vi "Trajectory Example.vi"() -> ()   [LabVIEW 2019]
uses:
  Typedef/Trajectory.ctl
  Typedef/Trajectory State.ctl
  Geometry/Typedef/Pose2d.ctl
  Geometry/Typedef/Translation2d.ctl
  Geometry/Typedef/Rotation2d.ctl
  Typedef/Differential Drive Constants.ctl
  Typedef/Differential Drive Constraints.ctl
panel:
  in  "Constraints":T1={"maxVoltage"=10.0, "maxVelocity"=5.0, "maxAccel"=10.0}
  in  "Constants":T2={"ks"=0.2, "kv"=0.18, "ka"=0.1, "trackwidth"=1.0}
  in  "Waypoints":T3[](array[typedef])=[{"Translation2d"={"x"=0.0, "y"=0.0}, "Rotation2d"={"Theta"=0.0}}, {"Translation2d"={"x"=1.0, "y"=1.0}, "Rotation2d"={"Theta"=1.0}}, {"Translation2d"={"x"=3.0, "y"=4.0}, "Rotation2d"={"Theta"=2.0}}]
  out "states":T6
  out "XY Graph 2":cluster{dbl[], dbl[]}(graph)
  out "XY Graph":cluster{dbl[], dbl[]}[](graph)
  out "Total Time Seconds":dbl
  out "error out":errorcluster
  in  "error in (no error)":errorcluster
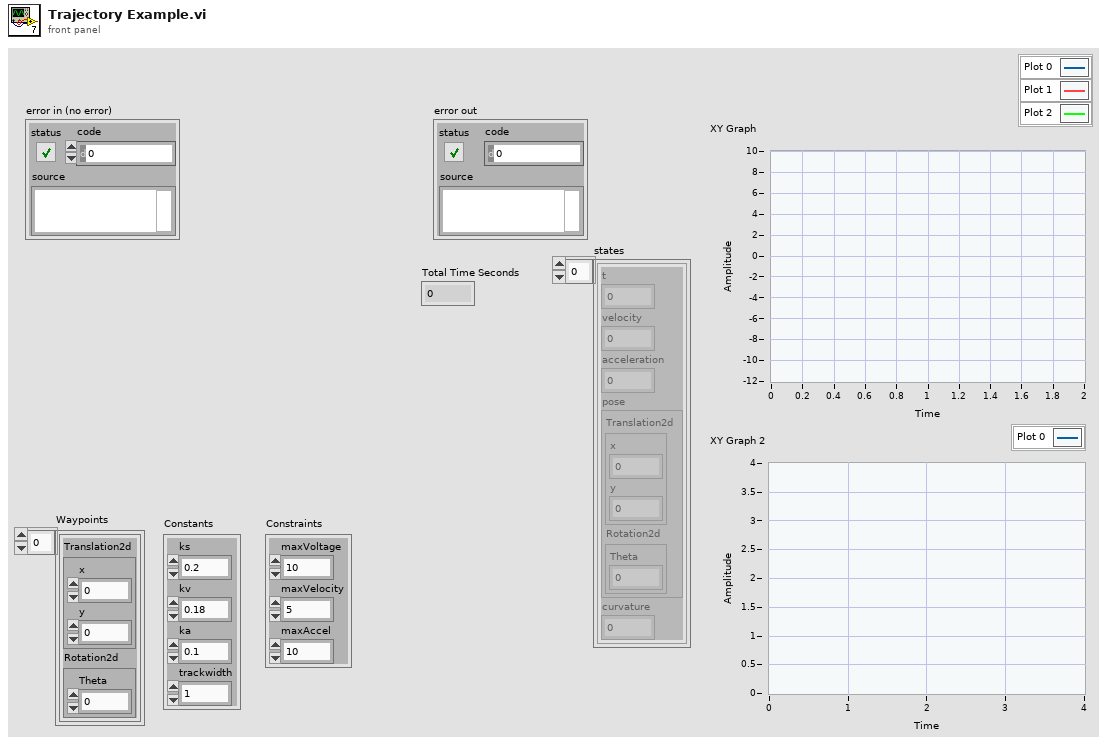
[diagram p1: front panel]
types:
  T1 = typedef "Differential Drive Constraints.ctl" = cluster{"maxVoltage":dbl, "maxVelocity":dbl, "maxAccel":dbl}
  T2 = typedef "Differential Drive Constants.ctl" = cluster{"ks":dbl, "kv":dbl, "ka":dbl, "trackwidth":dbl}
  T3 = typedef "Pose2d.ctl" = cluster{"Translation2d":T4, "Rotation2d":T5}
  T4 = typedef "Translation2d.ctl" = cluster{"x":dbl, "y":dbl}
  T5 = typedef "Rotation2d.ctl" = cluster{"Theta":dbl}
  T6 = typedef "Trajectory.ctl" = T7[]
  T7 = typedef "Trajectory State.ctl" = cluster{"t":dbl, "velocity":dbl, "acceleration":dbl, "pose":T3, "curvature":dbl}
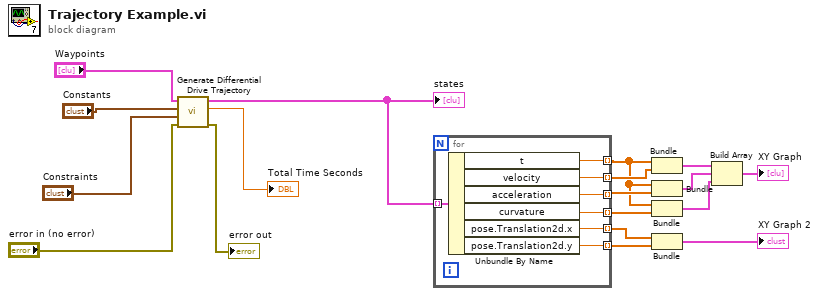
[diagram p0: block diagram]
diagram:
  n1 = call "Generate Differential Drive Trajectory.vi"("error in (no error)"="error in (no error)", "Constraints"="Constraints", "Constants"="Constants", "Waypoints"="Waypoints") -> ("error out"=→"error out":errorcluster, "Total Time Seconds"=→"Total Time Seconds":dbl, "states"=w1:T7[])  [unwired: 5 in]
  "states" <- w1
  n2 = for {
    tunnel: w1 -> [w25] mode=indexing
    tunnel: [w24] -> w17 mode=indexing
    tunnel: [w23] -> w16 mode=indexing
    tunnel: [w22] -> w12 mode=indexing
    tunnel: [w21] -> w15 mode=indexing
    tunnel: [w20] -> w14 mode=indexing
    tunnel: [w19] -> w13 mode=indexing
    n3 = Unbundle By Name(w25) -> ("t"=w22:dbl, "velocity"=w21:dbl, "acceleration"=w20:dbl, "curvature"=w19:dbl, "pose.Translation2d.x"=w24:dbl, "pose.Translation2d.y"=w23:dbl)
  }
  n4 = Bundle(w12, w15) -> (w9:cluster{dbl[], dbl[]})  [unwired: 1 in]
  n5 = Bundle(w12, w14) -> (w10:cluster{dbl[], dbl[]})  [unwired: 1 in]
  n6 = Bundle(w12, w13) -> (w11:cluster{dbl[], dbl[]})  [unwired: 1 in]
  n7 = Bundle(w17, w16) -> (→"XY Graph 2":cluster{dbl[], dbl[]})  [unwired: 1 in]
  n8 = Build Array(w9, w10, w11) -> (→"XY Graph":cluster{dbl[], dbl[]}[])
